vi "Value Change.vi"(5 "object ref in":T2, 8 "error in (no error)":errorcluster, 9 "old values":string[][](array[string]), 10 "Table Change":T1, 11 "List Box Enum Column in":refnum<class "List Box Enum Column.lvclass">) -> (0 "error out":errorcluster, 3 "List Box Enum Column out":refnum<class "List Box Enum Column.lvclass">)   [LabVIEW 2013, in "Table Manager.lvlib" / "List Box Enum Column.lvclass"]
uses:
  List Box Enum Column.lvclass
  Table Manager/object ref.ctl
  Configuration Editor/Classes/Engine Parent/Engine Parent Editor Node.lvclass
  Configuration Editor/Classes/Module editor node/module editor node.lvclass
  Table Manager/Cell Change.ctl
  Column/Column.lvclass/Column.ctl
  Column/Read Call Back VI.vi
  Table Manager/Table Manager.lvclass
  Table Manager.lvlib
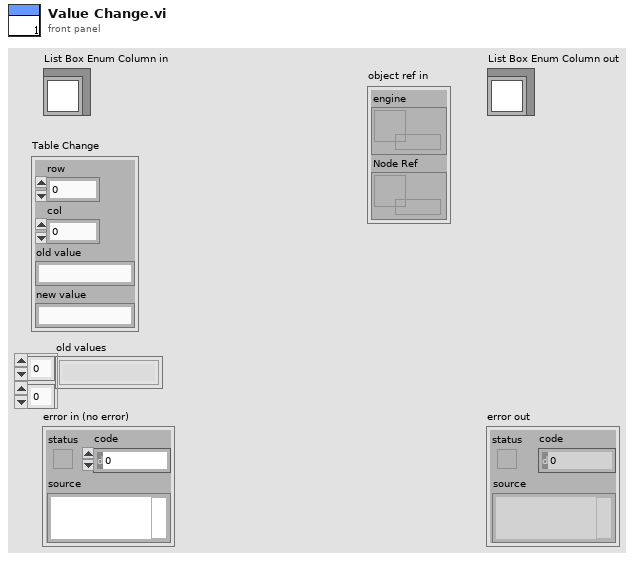
[diagram p1: front panel]
types:
  T1 = typedef "Table Manager.lvlib/Cell Change.ctl" = cluster{"row":i32, "col":i32, "old value":string, "new value":string}
  T2 = typedef "Table Manager.lvlib/Table Manager.lvclass/object ref.ctl" = cluster{"engine":refnum<data-value>, "Node Ref":refnum<data-value>}
  T3 = typedef "Table Manager.lvlib/Table Manager.lvclass/Call Back Ref Type Def.ctl" = refnum<vi>
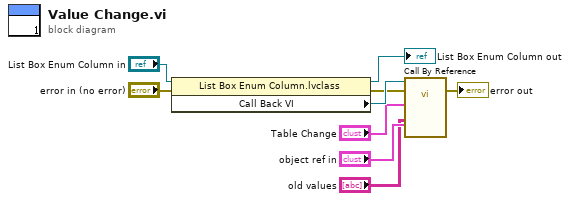
[diagram p0: block diagram]
diagram:
  n1 = property class="List Box Enum Column.lvclass"(reference="List Box Enum Column in", error in="error in (no error)") -> (reference out=→"List Box Enum Column out":refnum<class "List Box Enum Column.lvclass">, error out=w7:errorcluster, "Call Back VI"=w9:T3)
  n2 = call-by-ref "?"(reference=w9, error in=w7, "Variant"="object ref in", "old values"="old values", "Cluster"="Table Change") -> (error out=→"error out":errorcluster)  [unwired: 8 in, 2 out]
